vi "Set Configuration.vi"(6 "Value":bool, 8 "error in (no error)":errorcluster, 9 "Direction (F=Output,T=Input)":bool, 10 "Pin Mark":u8, 11 "IO-4 Bricklet in":refnum<class "IO-4 Bricklet.lvclass">) -> (0 "error out":errorcluster, 3 "IO-4 Bricklet out":refnum<class "IO-4 Bricklet.lvclass">)   [LabVIEW 2011, in "Tinkerforge.lvlib" / "IO-4 Bricklet.lvclass"]
doc: "This VI configures the value and direction of the specified pins. Possible directions are “i” and “o” for input and output.\n\nIf the direction is configured as output, the value is either high or low (set as true or false).\n\nIf the direction is configured as output, the value is either pull up or default (set as true or false).\n\nFor example:\n\n (15, ‘i’, true) will set all pins of as input pull up.\n (8, ‘i’, false) will set pin 3 of as input default (floating if nothing is connected).\n (3, ‘o’, false) will set pins 0 and 1 as output low.\n (4, ‘o’, true) will set pin 2 of as output high."
uses:
  IO-4 Bricklet.lvclass
  Device/Device.lvclass
  IP Connection/IP Connection.lvclass
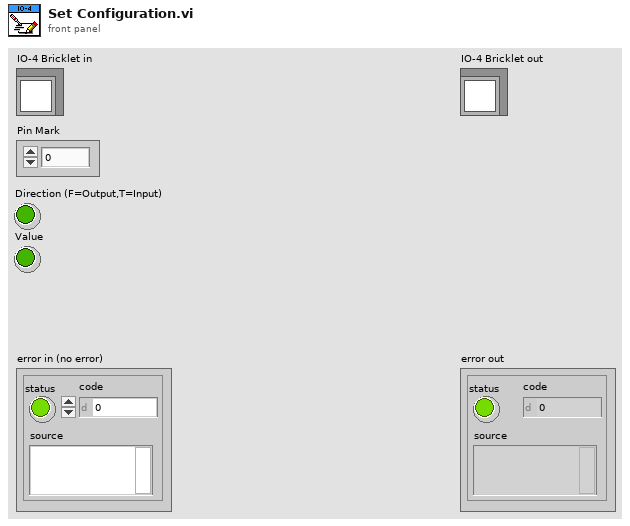
[diagram p1: front panel]
types:
  T1 = enum16{"big-endian, network order", "native, host order", "little-endian"}
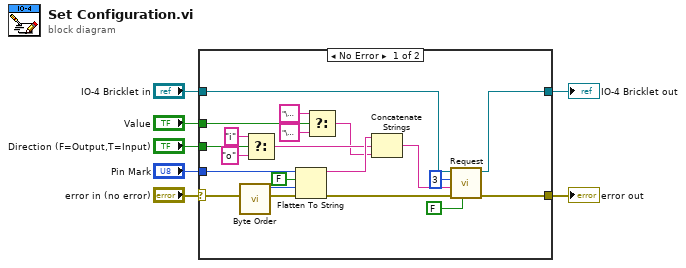
[diagram p0: block diagram]
diagram:
  n1 = case shown="No Error" "error in (no error)" {
    selector: "error in (no error)" -> [w22 w29]
    tunnel: [w23 w29] -> w6
    tunnel: [w26 w28] -> w4
    tunnel: "IO-4 Bricklet in" -> [w27 w28]
    tunnel: "Pin Mark" -> [w20 _]
    tunnel: "Direction (F=Output,T=Input)" -> [w17 _]
    tunnel: "Value" -> [w12 _]
    frame No Error {
      n2 = call "Byte Order.vi"() -> ("byte order (2:little-endian)"=w18:T1)  [unwired: 11 in]
      n3 = Select(t="i", s=w17, f="o") -> (s? t:f=w10:string)
      n4 = Flatten To String(anything=w20, prepend array or string size? (T)=FALSE, byte order (0:big-endian, network order)=w18, error in (no error)=w22) -> (data string=w11:string, error out=w21:errorcluster)  [unwired: 1 out]
      n5 = Select(t="\u0001", s=w12, f="\u0000") -> (s? t:f=w9:string)
      n6 = Concatenate Strings(w11, w10, w9) -> (w8:string)
      n7 = call "Request.vi"("Response"=FALSE, "error in (no error)"=w21, "Data"=w8, "Function ID"=u8 3, "Device in"=w27) -> ("error out"=w23:errorcluster, "Device out"=w26:refnum<class "IO-4 Bricklet.lvclass">)  [unwired: 2 in, 3 out]
    }
    frame Error {
    }
  }
  "error out" <- w6
  "IO-4 Bricklet out" <- w4
